vi "Update Target Conditional.vi"(8 "error in (no error)":errorcluster, 11 "Time Target (s)":dbl) -> (0 "error out":errorcluster)   [LabVIEW 2019]
uses:
  CLD 2 Time Mode.ctl
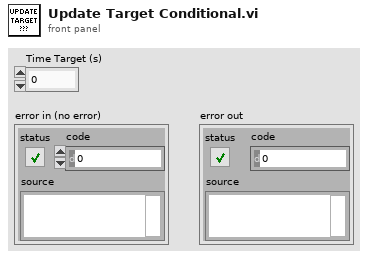
[diagram p1: front panel]
types:
  T1 = typedef "CLD 2 Time Mode.ctl" = enum16{"Reset", "Read Status", "Auto Reset and Status", "Update Target"}
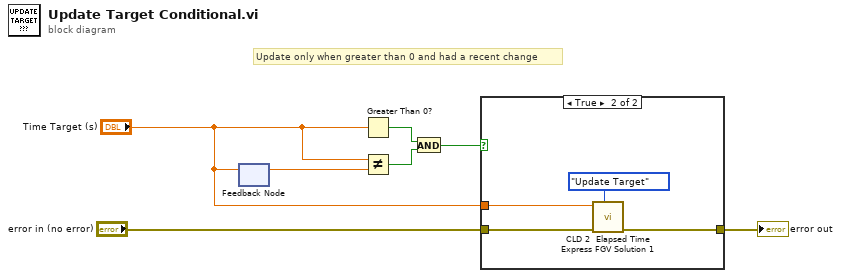
[diagram p0: block diagram]
diagram:
  # "Update only when greater than 0 and had a recent change"
  n1 = feedback-in #1("Time Target (s)") -> ()
  n2 = feedback #1() -> (w5:dbl)  [unwired: 1 in]
  n3 = Greater Than 0?(x="Time Target (s)") -> (x > 0?=w4:bool)
  n4 = Not Equal?(x="Time Target (s)", y=w5) -> (x != y?=w3:bool)
  n5 = And(x=w4, y=w3) -> (x .and. y?=w2:bool)
  n6 = case shown="True" w2 {
    tunnel: "error in (no error)" -> [w8 w12]
    tunnel: [w8 w11] -> w6
    tunnel: "Time Target (s)" -> [_ w9]
    frame False {
    }
    frame True {
      n7 = call "CLD 2  Elapsed Time Express FGV Solution 1.vi"("Timer  Mode"=CLD_2_Time_Mode."Update Target", "error in (no error)"=w12, "Time Target (s)"=w9) -> ("error out"=w11:errorcluster)  [unwired: 6 in, 2 out]
    }
  }
  "error out" <- w6
